vi "Actor Core.vi"(8 "error in":errorcluster, 11 "Nested in":refnum<class "UI_Left_Right.lvclass">) -> (0 "error out":errorcluster, 3 "Actor out":refnum<class "Actor.lvclass">)   [LabVIEW 2021, in "UI_Left_Right.lvclass"]
doc: "(<B>Filename</B>: Actor Framework.lvlib:Actor.lvclass:Actor Core.vi)\n\nReceives messages to the actor, reacts to them, and initiates any error handling that may shut the actor down.\n\nDescendant classes may override this VI to append parallel tasks for the actor to complete while it handles messages. Overrides use the Call Parent Method node."
uses:
  UI_Left_Right.lvclass
  <vilib>/ActorFramework/Actor/Actor.lvclass
  <vilib>/ActorFramework/Stop Msg/Stop Msg.lvclass
  C:/Program Files (x86)/National Instruments/LabVIEW 2021/user.lib/John_Lib/AbstractActorTemplate/AbstractActorTemplate/UIActorTop.lvclass
  C:/Program Files (x86)/National Instruments/LabVIEW 2021/vi.lib/ActorFramework/Actor/Actor.lvclass
  Z:/UTP_2023/Source_SequenceEdit - Copy/UI_Left_Right/UI_Left_Right.lvclass
  <userlib>/John_Lib/AbstractActorTemplate/AbstractActorTemplate/UIActorTop.lvclass
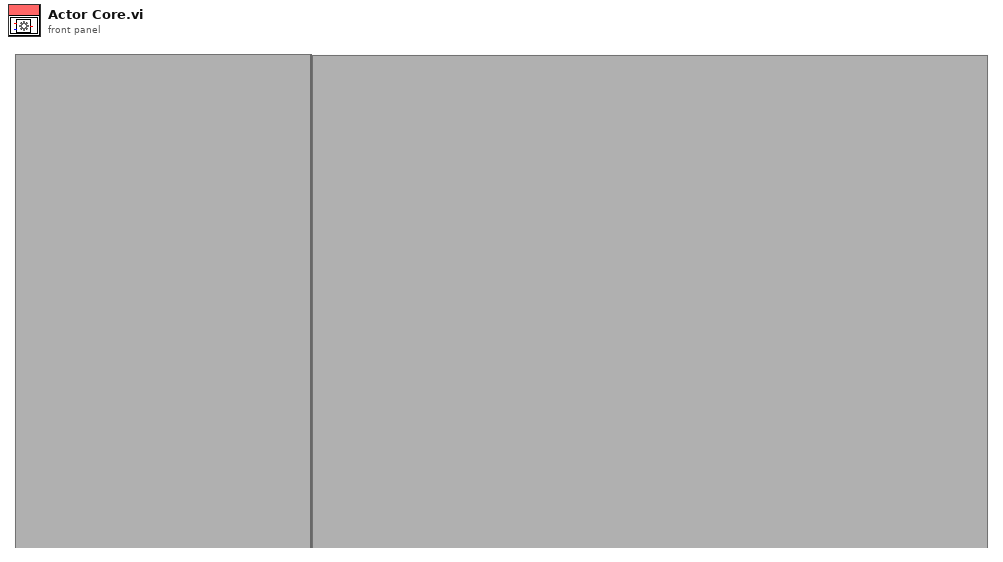
[diagram p1: front panel]
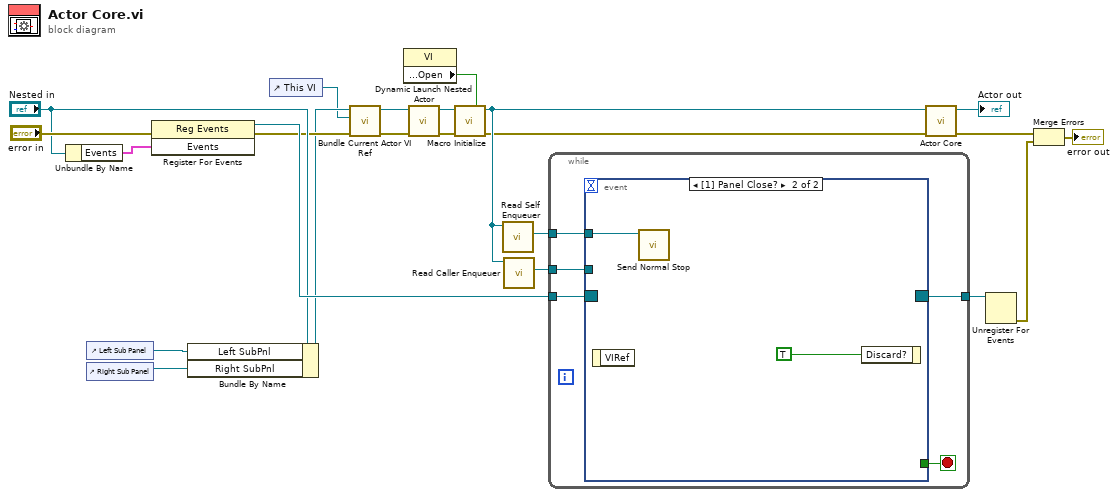
[diagram p0: block diagram]
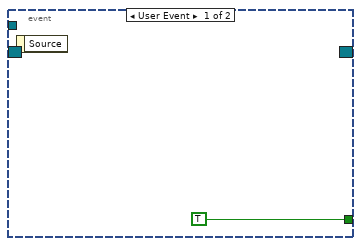
[diagram p2: hidden frame]
diagram:
  n1 = Unbundle By Name("Nested in") -> ("Events"=w21:cluster{"Stop":refnum<user-event>})
  n2 = control-ref of="Left Sub Panel"() -> (w5:refnum<vi>)
  n3 = control-ref of="Right Sub Panel"() -> (w4:refnum<vi>)
  n4 = register-events ("Main Register for Events")(error in="error in", w21) -> (reference out=w22:refnum<event-registration>, error out=w8:errorcluster)  [unwired: 1 in]
  n5 = Bundle By Name(cluster="Nested in", "Left SubPnl"=w5, "Right SubPnl"=w4) -> (w6:refnum<class "UI_Left_Right.lvclass">)
  n6 = control-ref of="This VI"() -> (w1:refnum<vi>)
  n7 = call <userlib>:"Bundle Current Actor VI Ref.vi"("error in (no error)"=w8, "This VI"=w1, "UI ActorTop in"=w6) -> ("error out"=w7:errorcluster, "UI ActorTop out"=w9:refnum<class "UI_Left_Right.lvclass">)  [unwired: 6 in, 1 out]
  n8 = property class="VI"() -> ("Front Panel.Open"=w17:bool)  [unwired: 2 in, 2 out]
  n9 = call-dynamic "Dynamic Launch Nested Actor.vi"("error in (no error)"=w7, "UI ActorTop in"=w9) -> ("error out"=w18:errorcluster, "UI ActorTop out"=w19:refnum<class "UI_Left_Right.lvclass">)  [unwired: 8 in]
  n10 = call-dynamic "Macro Initialize.vi"("Front Panel Window:Open"=w17, "error in (no error)"=w18, "UI ActorTop in"=w19) -> ("error out"=w11:errorcluster, "UI ActorTop out"=w15:refnum<class "UI_Left_Right.lvclass">)  [unwired: 7 in]
  n11 = call <vilib>:"Read Self Enqueuer.vi"("Actor"=w15) -> ("Self Enqueuer"=w3:refnum<class "Message Enqueuer.lvclass">)  [unwired: 10 in]
  n12 = call <vilib>:"Read Caller Enqueuer.vi"("Actor"=w15) -> ("Caller Enqueuer"=w2:refnum<class "Message Enqueuer.lvclass">)  [unwired: 10 in]
  n13 = while {
    tunnel: w22 -> [w28]
    tunnel: [w26] -> w20
    tunnel: w3 -> [w25]
    tunnel: w2 -> [w24]
    stop <- w27 stop-if-true
    n14 = event "UI Events" shown="[1] Panel Close?" {
      selector: w28 -> [_ _]
      dyn-events: [_ _] -> w26
      timeout: _ -> [_ _]
      tunnel: [TRUE _] -> w27
      tunnel: w25 -> [_ w30]
      tunnel: w24 -> [_ _]
      event User Event {
        n15 = event-data() -> ()  [unwired: 1 in, 1 out]
      }
      event Panel Close? {
        n16 = event-data() -> ()  [unwired: 1 in, 1 out]
        n17 = call <vilib>:"Send Normal Stop.vi"("Message Enqueuer"=w30) -> ()  [unwired: 10 in, 1 out]
        n18 = event-data("Discard?"=TRUE) -> ()  [unwired: 1 in, 1 out]
      }
    }
  }
  n19 = call-parent "Actor Core.vi"("error in"=w11, "Actor in"=w15) -> ("error out"=w13:errorcluster, "Actor out"=→"Actor out":refnum<class "Actor.lvclass">)  [unwired: 8 in]
  n20 = Unregister For Events(event registration refnum=w20) -> (error out=w14:errorcluster)  [unwired: 1 in]
  n21 = Merge Errors(w13, w14) -> (→"error out":errorcluster)
